vi "DQ subVI.vi"(9 "window (h)":i32, 11 "XY-data":cluster{"X-array":dbl[], "Y-array":dbl[]}) -> (3 "XY-data out":cluster{"X-array":dbl[], "Y-array":dbl[]})   [LabVIEW 2019, in "xy_utilities.lvlib"]
uses:
  xy_utilities.lvlib
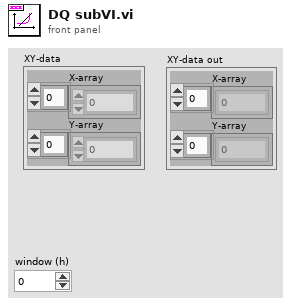
[diagram p1: front panel]
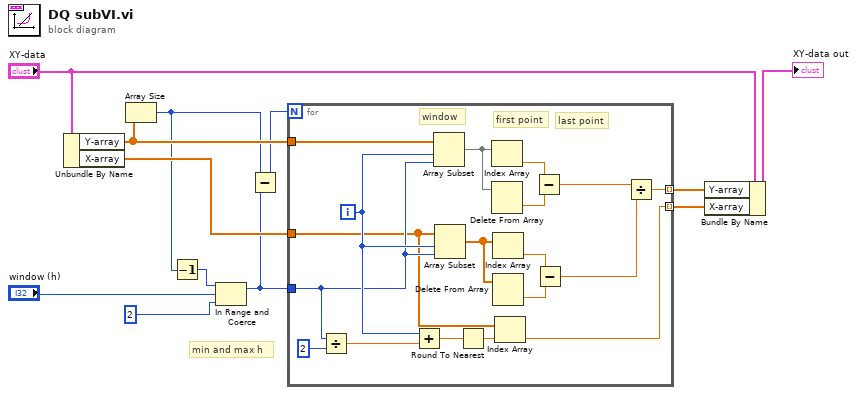
[diagram p0: block diagram]
diagram:
  # "min and max h"
  n1 = Unbundle By Name("XY-data") -> ("Y-array"=w12:dbl[], "X-array"=w8:dbl[])
  n2 = Array Size(array=w12) -> (size(s)=w1:i32)
  n3 = Decrement(x=w1) -> (x-1=w2:i32)
  n4 = In Range and Coerce(upper limit=w2, x="window (h)", lower limit=2) -> (coerced(x)=w5:i32)  [unwired: 1 out]
  n5 = Subtract(x=w1, y=w5) -> (x-y=w7:i32)
  n6 = for {
    N: w7 -> [_]
    tunnel: w12 -> [w30]
    tunnel: w8 -> [w13]
    tunnel: w5 -> [w14]
    tunnel: [w23] -> w10 mode=indexing
    tunnel: [w16] -> w6 mode=indexing
    i -> [w20]
    # "last point"
    # "first point"
    # "window"
    n7 = Divide(x=w14, y=2) -> (x/y=w18:dbl)
    n8 = Add(x=w20, y=w18) -> (x+y=w17:dbl)
    n9 = Array Subset(array=w30, index=w20, length=w14) -> (w29:dbl[])
    n10 = Array Subset(array=w13, index=w20, length=w14) -> (w24:dbl[])
    n11 = Round To Nearest(number=w17) -> (nearest integer value=w15:dbl)
    n12 = Index Array(array=w29) -> (element=w28:dbl)  [unwired: 1 in]
    n13 = Delete From Array(array=w29) -> (deleted portion=w27:dbl)  [unwired: 2 in, 1 out]
    n14 = Index Array(array=w24) -> (element=w25:dbl)  [unwired: 1 in]
    n15 = Delete From Array(array=w24) -> (deleted portion=w26:dbl)  [unwired: 2 in, 1 out]
    n16 = Index Array(array=w13, index=w15) -> (element=w16:dbl)
    n17 = Subtract(x=w28, y=w27) -> (x-y=w22:dbl)
    n18 = Subtract(x=w25, y=w26) -> (x-y=w21:dbl)
    n19 = Divide(x=w22, y=w21) -> (x/y=w23:dbl)
  }
  n20 = Bundle By Name(cluster="XY-data", "Y-array"=w10, "X-array"=w6) -> (→"XY-data out":cluster{"X-array":dbl[], "Y-array":dbl[]})
